vi "GUI_update.vi"(0 "reference":refnum<class "OSA.lvclass">, 5 "error in (no error)":errorcluster, 6 "ctrl refs":T1, 7 "y unit":T3, 9 "spectrum x unit":T2) -> (10 "acq stopped":bool, 14 "duplicate reference":refnum<class "OSA.lvclass">, 15 "X interferogram":cluster{"A":dbl, "B":dbl, "B-A":dbl} {"B-A" format="%^.2e"; "B" format="%.2f"; "A" format="%.2f"}, 16 "Y interferogram":cluster{"A":dbl, "B":dbl, "B-A":dbl} {"B-A" format="%^.2e"; "B" format="%.2f"; "A" format="%.2f"}, 17 "X spectrum":cluster{"A":dbl, "B":dbl, "B-A":dbl} {"B-A" format="%^.2e"; "B" format="%.2f"; "A" format="%.2f"}, 18 "Y spectrum":cluster{"A":dbl, "B":dbl, "B-A":dbl} {"B-A" format="%^.2e"; "B" format="%.2f"; "A" format="%.2f"}, 19 "error out":errorcluster)   [LabVIEW 2010, in "OSA.lvclass"]
doc: "Reads the contents of a <B>Thorlabs_OSA_64</B> object.\n\n[GOOP 1.0]"
uses:
  OSA.lvclass
  y_unit_GUI.ctl
  typeDef/spectrum_x_unit.ctl
  ctrlRefs.ctl
  typeDef/acq_dataType.ctl
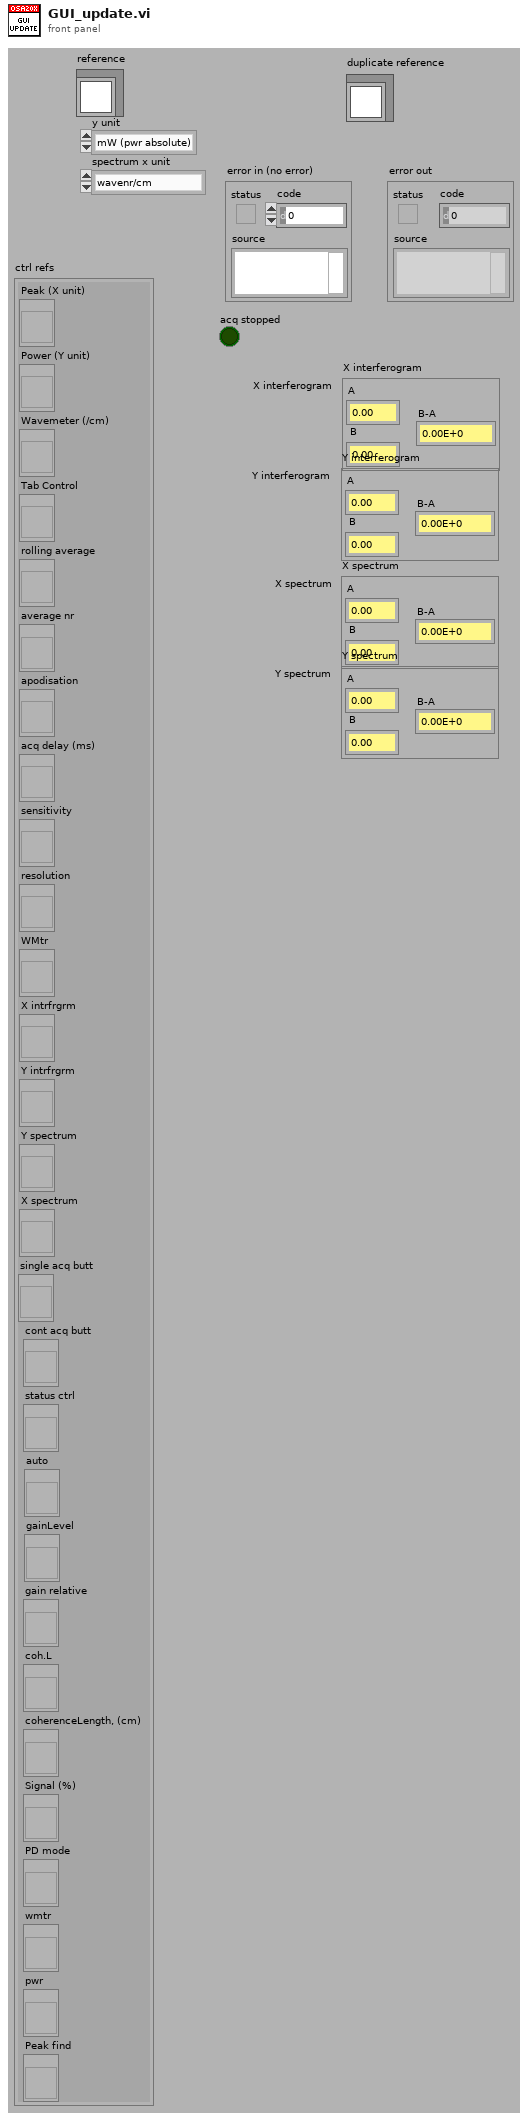
[diagram p1: front panel]
types:
  T1 = typedef "OSA.lvclass/ctrlRefs.ctl" = cluster{"Peak (X unit)":refnum<vi>, "Power (Y unit)":refnum<vi>, "Wavemeter (/cm)":refnum<vi>, "Tab Control":refnum<vi>, "rolling average":refnum<vi>, "average nr":refnum<vi>, "apodisation":refnum<vi>, "acq delay (ms)":refnum<vi>, "sensitivity":refnum<vi>, "resolution":refnum<vi>, "WMtr":refnum<vi>, "X intrfrgrm":refnum<vi>, "Y intrfrgrm":refnum<vi>, "Y spectrum":refnum<vi>, "X spectrum":refnum<vi>, "single acq butt":refnum<vi>, "cont acq butt":refnum<vi>, "status ctrl":refnum<vi>, "auto":refnum<vi>, "gainLevel":refnum<vi>, "gain relative":refnum<vi>, "coh.L":refnum<vi>, "coherenceLength, (cm)":refnum<vi>, "Signal (%)":refnum<vi>, "PD mode":refnum<vi>, "wmtr":refnum<vi>, "pwr":refnum<vi>, "Peak find":refnum<vi>}
  T2 = typedef "OSA.lvclass/spectrum_x_unit.ctl" = enum16{"wavenr/cm", "THz", "eV", "nm_air", "nm_vac"}
  T3 = typedef "OSA.lvclass/y_unit_GUI.ctl" = enum16{"mW (pwr absolute)", "dBm (pwr absolute)"}
  T4 = enum8{"Enabled", "Disabled", "Disabled and Grayed Out"}
  T5 = enum16{"cool: better sensitivity/noise floor", "warm: extended wl range"}
  T6 = typedef "OSA.lvclass/acq_dataType.ctl" = enum16{"none", "interferogram", "spectrum"}
  T7 = typedef "OSA.lvclass/ObjectAttributes.ctl" = cluster{"Stop":bool, "dataType":T6, "spectrometerIdx":u16, "buffer size interferogram":i32, "interferogram":cluster{"new":bool, "plot_x_ min":sgl, "plot_x_max":sgl, "plot_y_min":sgl, "plot_y_max":sgl, "Graph Intrfrgrm":T8, "timeStamp":u32, "signal (%)":dbl, "traces":cluster{"idx":u32, "broadBand":bool, "monoChromatic":bool, "peakToPeakSignal":dbl, "peakToPeakPos":dbl}[], "traces idx last":i32}, "spectrum":cluster{"new":bool, "plot_x_min":sgl, "plot_x_max":sgl, "plot_unit_x":T2, "plot_unit_y":T9, "plot_y_min":sgl, "plot_y_max":sgl, "Graph Spectrum":T8, "timeStamp":u32, "X_VAL_OPTIONS":enum16{"MIN_MAX", "ARRAY"}, "traces":cluster{"idx":u32}[], "traces idx last":i32}, "Thorlabs_OSA_64.lvclass:queue_action.ctlqueue ref":refnum<queue>, "action":T10, "plot zoom step":dbl, "buffer semaphore":T11, "acq stopped":bool, "dataType active":T6, "temperature (degr C)":sgl, "pressure (hPa)":sgl, "rel humidity (%)":sgl, "settings":cluster{"resolution":T12, "sensitivity":T13, "Average":bool, "average nr":u32, "apodisation":T14, "acq delay (ms)":u32, "airMesure":T15, "wmtr on":bool, "intfgrm_smooth_width":u16, "intfgrm_smooth_nrOfPasses":u16, "intfgrm_smooth":T16, "phaseCorrection":T17, "zeroFill":u8, "spectr_smooth":T16, "spectr_smooth_width":u16, "spectr_smooth_nrOfPasses":u16, "resolution (/cm)":sgl, "REF wavelength, (nm)":dbl, "gain_idx":u16, "gainAuto":bool, "gain_relative":dbl, "PD sensitivity mode":T18, "PD senseMode implemented":bool, "SensorTemperature implemented":bool, "SensorPressure implemented":bool, "SensorHumidity implemented":bool}, "peaks position":sgl[], "peaks width":sgl[], "peaks height":sgl[], "peaks max nr":u32, "peaks latest nr":i32, "peaks new":bool, "power":dbl, "power new":bool, "path":string, "wavelength (WNr)":dbl, "wavelength new":bool, "buffer size spectrum":i32, "status":string, "VI reference":refnum<vi>, "funcPointer":u64, "libraryPointer":u64, "singleAcquisition":bool, "coherenceLength (cm)":dbl, "coherenceLength new":bool, "spectrometer model":string, "spectrometer serial nr":string, "peaks thld left":sgl[], "peaks thld right":sgl[], "coherenceLength error (cm)":dbl, "ADC bits":u16, "peaks position centroid":sgl[], "peaks height centroid":sgl[], "OSA series":T19, "channel index":u16}
  T8 = typedef "OSA.lvclass/graph_intensity.ctl" = refnum<vi>
  T9 = typedef "OSA.lvclass/y_unit.ctl" = enum16{"ADC counts", "dBm pwr absolute", "dBm pwr density", "mW pwr absolute", "mW pwr density"}
  T10 = typedef "OSA.lvclass/queue_action.ctl" = enum16{"none", "stop", "GUI_plotInterferogram", "GUI_plotSpectrum", "GUI_plotInterferogramRescale", "GUI_plotSpectrumRescale", "GUI_plotInterferogramReset", "GUI_plotSpectrumReset", "GUI_plotInterferogramAutoScaleY", "GUI_plotSpectrumAutoScaleY", "GUI_plotInterferogramZoomOut", "GUI_plotSpectrumZoomOut", "GUI_plotInterferogramPane", "GUI_plotSpectrumPane", "GUI_plotInterferogramZoomMouse", "GUI_plotSpectrumZoomMouse", "ENVIRONMENT temperature", "ENVIRONMENT pressure", "MODE_resolution set", "MODE_resolution get", "MODE_sensitivity set", "MODE_sensitivity get", "MODE_PDTemperature set", "MODE_PDTemperature get", "REBOOT/RESET firmware", "ACQASYNC_acquireSingleSpectrum", "ACQASYNC_continuous start", "ACQASYNC_continuous stop\n", "ACQASYNC_get last interferogram", "ACQASYNC_get last spectrum", "ACQASYNC_get last waveNr", "ACQOPT_interferogram smoothing set", "ACQOPT_interferogram smoothing get", "ACQOPT_spectrum smoothing set", "ACQOPT_spectrum smoothing get", "ACQOPT_apodisation type set", "ACQOPT_apodisation type get", "ACQOPT_phase correction type set", "ACQOPT_phase correction type get", "ACQOPT_acqIntervall_set", "ACQOPT_acqIntervall_get", "ACQOPT_average spectrum set", "ACQOPT_average spectrum get", "ACQOPT_rolling average set", "ACQOPT_rolling average get", "ACQOPT_zero fill factor set", "ACQOPT_zero fill factor get", "ACQOPT_cycle counting set", "ACQOPT_cycle counting get", "ACQOPT_air measure option set", "ACQOPT_air measure option get", "ACQOPT_gainLevel auto get", "ACQOPT_gainLevel auto set", "ACQOPT_gainLevel get", "ACQOPT_gainLevel set", "ACQOPT_getAll", "INSTRUMENT_PROPERTY_range_WaveNr_min", "INSTRUMENT_PROPERTY_range_WaveNr_max", "INSTRUMENT_PROPERTY_reference_wavelength_cm^-1", "INSTRUMENT_PROPERTY_samplesPerRefPeriod", "INSTRUMENT_PROPERTY_resolution_waveNrPercm", "INSTRUMENT_PROPERTY_availableGainLevels", "INSTRUMENT_PROPERTY_status", "CONVERT", "ANALYSE_POWER", "ANALYSE_PEAKS", "ANALYSE_WAVELENGTH", "ANALYSE_SPECTRUM", "ANALYSE_INTERFEROGRAM", "ANALYSE_COHERENCE_LENGTH", "MATH", "MATH_power", "MATH_peaks", "FILE", "miscellaneous"}
  T11 = typedef "Semaphore RefNum" = refnum<k1>
  T12 = typedef "OSA.lvclass/resolution.ctl" = enum16{"low", "high"}
  T13 = typedef "OSA.lvclass/sensitivityMode.ctl" = enum16{"low", "low medium", "high medium", "high"}
  T14 = typedef "OSA.lvclass/apodisation.ctl" = enum16{"NONE", "NORTON_BEER_WEAK", "NORTON_BEER_MEDIUM", "NORTON_BEER_STRONG", "TRIANGULAR", "COSINE", "HANN", "HAMMING", "BLACKMANHARRIS3", "BLACKMANHARRIS4", "GAUSSIAN"}
  T15 = typedef "OSA.lvclass/airMeasure.ctl" = enum16{"TEMPERATURE", "PRESSURE"}
  T16 = typedef "OSA.lvclass/smoothing.ctl" = enum16{"NONE", "BINOMIAL", "SAVITSKY_GOLAY", "FOURIER", "MOVING_AVERAGE", "GAUSSIAN"}
  T17 = typedef "OSA.lvclass/phaseCorrection.ctl" = enum16{"NONE", "MERTZ", "FORMAN", "MERTZ_FILE", "FORMAN_FILE", "FUTURE COMP."}
  T18 = typedef "OSA.lvclass/PDTemperatureMode.ctl" = enum16{"cool: better sensitivity/noise floor", "warm: extended wl range"}
  T19 = typedef "OSA.lvclass/OSA_series.ctl" = enum16{"OSA200", "OSA300", "UNKNOWN"}
  T20 = typedef "Arrow Up.ctl" = bool
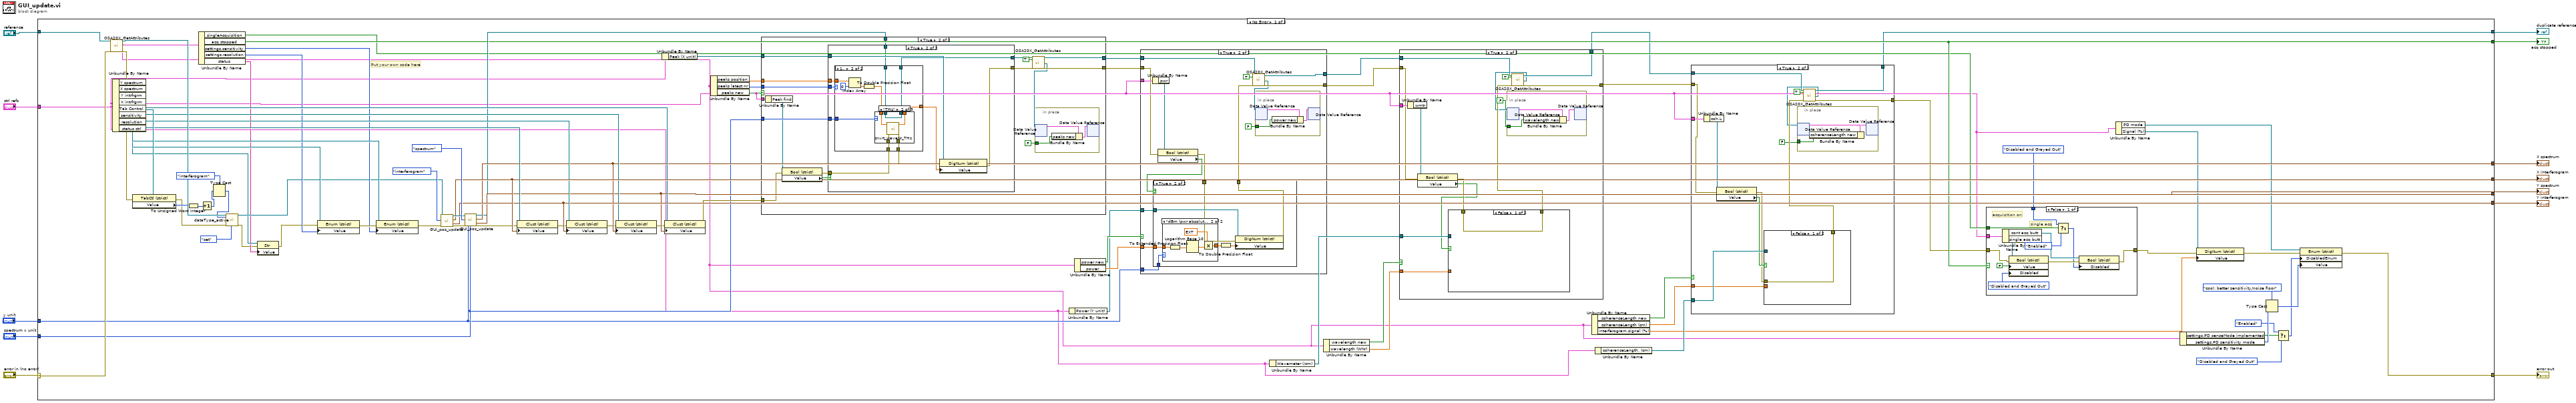
[diagram p0: block diagram]
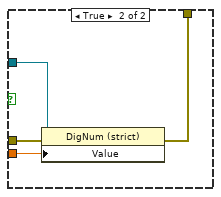
[diagram p3: hidden frame]
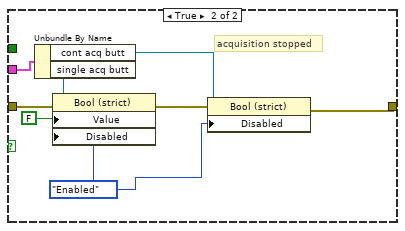
[diagram p4: hidden frame]
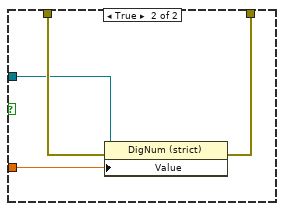
[diagram p6: hidden frame]
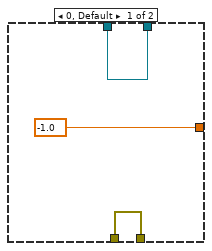
[diagram p12: hidden frame]
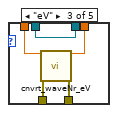
[diagram p14: hidden frame]
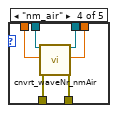
[diagram p15: hidden frame]
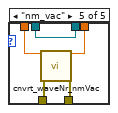
[diagram p16: hidden frame]
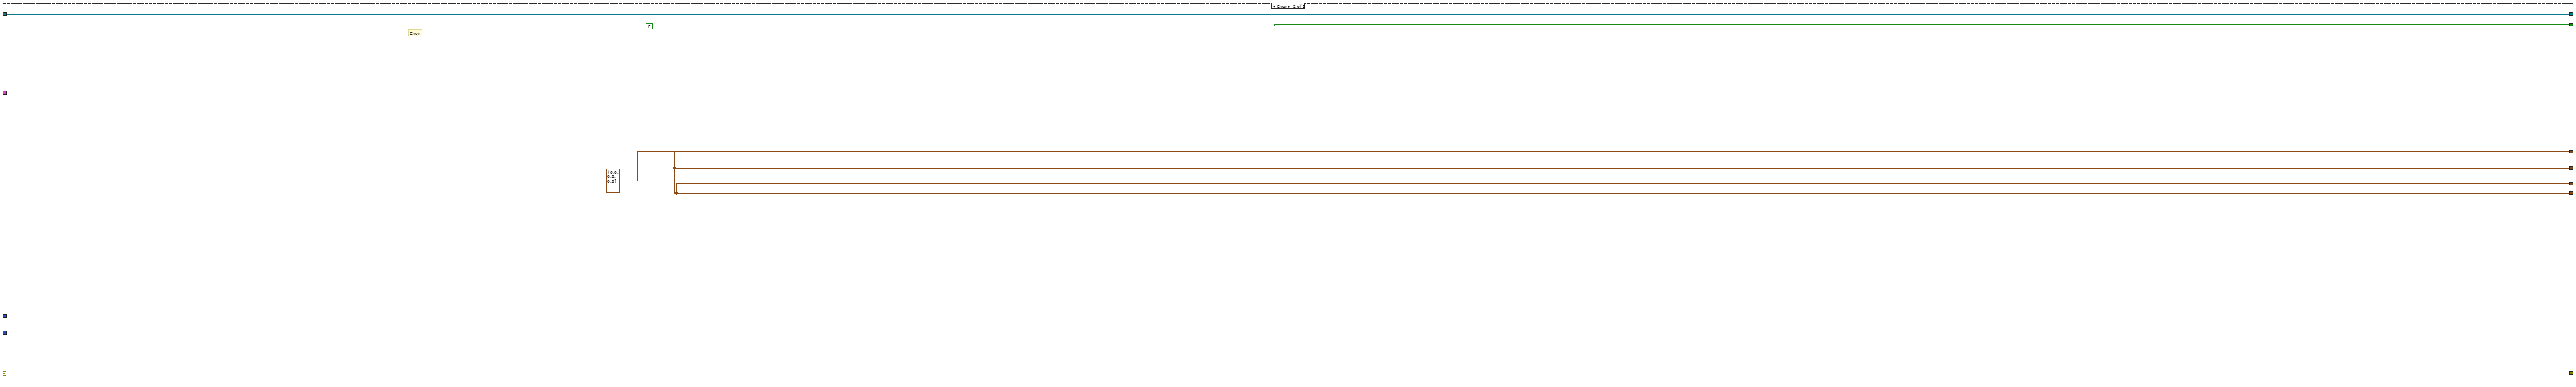
[diagram p17: hidden frame]
diagram:
  n1 = case shown="No Error" "error in (no error)" {
    selector: "error in (no error)" -> [w89 w270]
    tunnel: [w14 w270] -> w12
    tunnel: "reference" -> [w90 w271]
    tunnel: [w29 w271] -> w9
    tunnel: [w82 w269] -> w8
    tunnel: [w80 w269] -> w7
    tunnel: [w74 w269] -> w6
    tunnel: [w76 w269] -> w5
    tunnel: "spectrum x unit" -> [w58 _]
    tunnel: "y unit" -> [w50 _]
    tunnel: [w44 FALSE ("acq stopped")] -> w2
    tunnel: "ctrl refs" -> [w13 _]
    frame No Error {
      # "Put your own code here"
      n2 = call "OSA20X_GetAttributes.vi"("reference in"=w90, "error in (no error)"=w89) -> ("reference out"=w88:refnum<class "OSA.lvclass">, "Data"=w24:T7, "error out"=w71:errorcluster)  [unwired: 14 in, 1 out]
      n3 = Unbundle By Name(w13) -> ("Y spectrum"=w77:refnum<vi>, "X spectrum"=w78:refnum<vi>, "Y intrfrgrm"=w81:refnum<vi>, "X intrfrgrm"=w83:refnum<vi>, "Tab Control"=w84:refnum<vi>, "sensitivity"=w68:refnum<vi>, "resolution"=w67:refnum<vi>, "status ctrl"=w43:refnum<vi>)
      n4 = property class="TabCtl (strict)"(reference=w84, error in=w71) -> (error out=w85:errorcluster, "Value"=w87:enum32{"interferogram", "spectrum"})  [unwired: 1 out]
      n5 = To Unsigned Word Integer(number=w87) -> (unsigned 16bit integer=w86:u16)
      n6 = Unbundle By Name(w24) -> ("singleAcquisition"=w39:bool, "acq stopped"=w44:bool, "settings.sensitivity"=w65:T13, "settings.resolution"=w66:T12, "status"=w42:string)
      n7 = Increment(x=w86) -> (x+1=w36:u16)
      n8 = Type Cast(type=acq_dataType."interferogram" ("dataType active"), x=w36) -> (*(type *) &x=w35:T6)
      n9 = call "dataType_active.vi"("reference"=w88, "dataType active"=w35, "error in (no error)"=w85, "get/set"=enum16{"get", "set"}."set") -> ("duplicate reference"=w51:refnum<class "OSA.lvclass">, "error out"=w41:errorcluster)  [unwired: 13 in, 1 out]
      n10 = property class="Str"(reference=w43, error in=w41, "Value"=w42) -> (error out=w40:errorcluster)  [unwired: 1 out]
      n11 = property class="Enum (strict)"(reference=w67, error in=w40, "Value"=w66) -> (error out=w70:errorcluster)  [unwired: 1 out]
      n12 = property class="Enum (strict)"(reference=w68, error in=w70, "Value"=w65) -> (error out=w69:errorcluster)  [unwired: 1 out]
      n13 = call "GUI_pos_update.vi"("reference"=w51, "dataType"=acq_dataType."interferogram", "error in (no error)"=w69) -> ("reference out"=w92:refnum<class "OSA.lvclass">, "X"=w82:cluster{"A":dbl, "B":dbl, "B-A":dbl}, "Y"=w80:cluster{"A":dbl, "B":dbl, "B-A":dbl}, "error out"=w91:errorcluster)  [unwired: 13 in]
      n14 = call "GUI_pos_update.vi"("reference"=w92, "dataType"=acq_dataType."spectrum", "error in (no error)"=w91, "spectrum y unit"=w50, "spectrum x unit"=w58) -> ("reference out"=w59:refnum<class "OSA.lvclass">, "X"=w76:cluster{"A":dbl, "B":dbl, "B-A":dbl}, "Y"=w74:cluster{"A":dbl, "B":dbl, "B-A":dbl}, "error out"=w72:errorcluster)  [unwired: 11 in]
      n15 = property class="Clust (strict)"(reference=w83, error in=w72, "Value"=w82) -> (error out=w79:errorcluster)  [unwired: 1 out]
      n16 = property class="Clust (strict)"(reference=w81, error in=w79, "Value"=w80) -> (error out=w75:errorcluster)  [unwired: 1 out]
      n17 = property class="Clust (strict)"(reference=w78, error in=w75, "Value"=w76) -> (error out=w73:errorcluster)  [unwired: 1 out]
      n18 = Unbundle By Name(w13) -> ("Peak (X unit)"=w62:refnum<vi>)
      n19 = property class="Clust (strict)"(reference=w77, error in=w73, "Value"=w74) -> (error out=w64:errorcluster)  [unwired: 1 out]
      n20 = Unbundle By Name(w24) -> ("peaks position"=w60:sgl[], "peaks latest nr"=w61:i32, "peaks new"=w63:bool)
      n21 = case shown="True" w63 {
        tunnel: w64 -> [w197 w201]
        tunnel: w62 -> [_ w213]
        tunnel: w61 -> [_ w215]
        tunnel: w60 -> [_ w214]
        tunnel: [w197 w211] -> w52
        tunnel: w59 -> [w198 w205]
        tunnel: [w198 w210] -> w54
        tunnel: w58 -> [_ w209]
        tunnel: w13 -> [_ w203]
        frame False {
        }
        frame True {
          n22 = Unbundle By Name(w203) -> ("Peak find"=w202:refnum<vi>)
          n23 = property class="Bool (strict)"(reference=w202, error in=w201) -> (error out=w199:errorcluster, "Value"=w200:T20)  [unwired: 1 out]
          n24 = case shown="True" w200 {
            tunnel: w215 -> [_ w227]
            tunnel: w214 -> [_ w226]
            tunnel: w213 -> [_ w225]
            tunnel: [w216 w223] -> w212
            tunnel: w209 -> [_ w222]
            tunnel: w205 -> [w217 w221]
            tunnel: [w217 w220] -> w204
            tunnel: w199 -> [w216 w219]
            frame False {
            }
            frame True {
              n25 = case shown="1.." w227 {
                tunnel: w226 -> [_ w240]
                tunnel: [-1.0 ("Value") w237] -> w224
                tunnel: w222 -> [_ w236]
                tunnel: w219 -> [w229 w235]
                tunnel: [w229 w234] -> w218
                tunnel: w221 -> [w228 w233]
                tunnel: [w228 w232] -> w220
                frame 0, Default {
                }
                frame 1.. {
                  n26 = Index Array(array=w240, index=0) -> (element=w238:sgl)
                  n27 = To Double Precision Float(number=w238) -> (double precision float=w231:dbl)
                  n28 = case shown="\"THz\"" w236 {
                    tunnel: w231 -> [w241 w248 w253 w254 w264]
                    tunnel: [w241 w245 w250 w255 w261] -> w237
                    tunnel: w235 -> [w243 w247 w252 w259 w263]
                    tunnel: [w243 w246 w251 w258 w262] -> w234
                    tunnel: w233 -> [w242 w244 w249 w257 w260]
                    tunnel: [w242 w244 w249 w256 w260] -> w232
                    frame "wavenr/cm", Default {
                    }
                    frame "THz" {
                      n29 = call "cnvrt_waveNr_THz.vi"("waveNr"=w248, "error in (no error)"=w247) -> ("frequency (THz)"=w245:dbl, "error out"=w246:errorcluster)  [unwired: 16 in]
                    }
                    frame "eV" {
                      n30 = call "cnvrt_waveNr_eV.vi"("waveNr"=w253, "error in (no error)"=w252) -> ("energy (eV)"=w250:dbl, "error out"=w251:errorcluster)  [unwired: 16 in]
                    }
                    frame "nm_air" {
                      n31 = call "cnvrt_waveNr_nmAir.vi"("reference in"=w257, "waveNr"=w254, "error in (no error)"=w259) -> ("reference out"=w256:refnum<class "OSA.lvclass">, "wavelength (nmAir)"=w255:dbl, "error out"=w258:errorcluster)  [unwired: 14 in]
                    }
                    frame "nm_vac" {
                      n32 = call "cnvrt_waveNr_nmVac.vi"("waveNr"=w264, "error in (no error)"=w263) -> ("wavelength (nmVac)"=w261:dbl, "error out"=w262:errorcluster)  [unwired: 16 in]
                    }
                  }
                }
              }
              n33 = property class="DigNum (strict)"(reference=w225, error in=w218, "Value"=w224) -> (error out=w223:errorcluster)  [unwired: 1 out]
            }
          }
          n34 = call "OSA20X_GetAttributes.vi"("reference in"=w204, "OnlyGetDvrReference(False)"=TRUE, "error in (no error)"=w212) -> ("reference out"=w210:refnum<class "OSA.lvclass">, "DataRef"=w207:refnum<data-value>, "error out"=w211:errorcluster)  [unwired: 13 in, 1 out]
          n35 = in-place {
            in-place-border: FALSE ("peaks new") -> [w266]
            n36 = in-place-dvr #1(w207) -> (w267:T7)  [unwired: 1 out]
            n37 = Bundle By Name(cluster=w267, "peaks new"=w266) -> (w265:T7)
            n38 = in-place-dvr #1(w265) -> ()  [unwired: 2 out]
          }
        }
      }
      n39 = Unbundle By Name(w13) -> ("Power (Y unit)"=w53:refnum<vi>)
      n40 = Unbundle By Name(w24) -> ("power new"=w56:bool, "power"=w55:dbl)
      n41 = case shown="True" w56 {
        tunnel: w55 -> [_ w177]
        tunnel: w54 -> [w163 w179]
        tunnel: w53 -> [_ w178]
        tunnel: w52 -> [w164 w167]
        tunnel: [w164 w175] -> w45
        tunnel: w50 -> [_ w174]
        tunnel: [w163 w173] -> w46
        tunnel: w13 -> [_ w168]
        frame False {
        }
        frame True {
          n42 = Unbundle By Name(w168) -> ("pwr"=w169:refnum<vi>)
          n43 = property class="Bool (strict)"(reference=w169, error in=w167) -> (error out=w166:errorcluster, "Value"=w165:T20)  [unwired: 1 out]
          n44 = case shown="True" w165 {
            tunnel: w178 -> [_ w187]
            tunnel: w177 -> [_ w186]
            tunnel: [w180 w184] -> w176
            tunnel: w174 -> [_ w183]
            tunnel: w166 -> [w180 w181]
            frame False {
            }
            frame True {
              n45 = case shown="\"dBm (pwr absolute)\"" w183 {
                tunnel: w186 -> [w188 w191]
                tunnel: [w188 w192] -> w185
                frame "mW (pwr absolute)", Default {
                }
                frame "dBm (pwr absolute)" {
                  n46 = To Extended Precision Float(1:w191) -> (0:w190:ext)
                  n47 = Logarithm Base 10(1:w190) -> (0:w193:ext)
                  n48 = Multiply(x=ext 10.0, y=w193) -> (x*y=w192:ext)
                }
              }
              n49 = To Double Precision Float(number=w185) -> (double precision float=w182:dbl)
              n50 = property class="DigNum (strict)"(reference=w187, error in=w181, "Value"=w182) -> (error out=w184:errorcluster)  [unwired: 1 out]
            }
          }
          n51 = call "OSA20X_GetAttributes.vi"("reference in"=w179, "OnlyGetDvrReference(False)"=TRUE, "error in (no error)"=w176) -> ("reference out"=w173:refnum<class "OSA.lvclass">, "DataRef"=w171:refnum<data-value>, "error out"=w175:errorcluster)  [unwired: 13 in, 1 out]
          n52 = in-place {
            in-place-border: FALSE ("peaks new") -> [w195]
            n53 = in-place-dvr #2(w171) -> (w196:T7)  [unwired: 1 out]
            n54 = Bundle By Name(cluster=w196, "power new"=w195) -> (w194:T7)
            n55 = in-place-dvr #2(w194) -> ()  [unwired: 2 out]
          }
        }
      }
      n56 = Unbundle By Name(w13) -> ("Wavemeter (/cm)"=w47:refnum<vi>)
      n57 = Unbundle By Name(w24) -> ("wavelength new"=w49:bool, "wavelength (WNr)"=w48:dbl)
      n58 = case shown="True" w49 {
        tunnel: w48 -> [_ w152]
        tunnel: w46 -> [w139 w154]
        tunnel: w47 -> [_ w153]
        tunnel: w45 -> [w140 w143]
        tunnel: [w140 w150] -> w31
        tunnel: [w139 w149] -> w30
        tunnel: w13 -> [_ w144]
        frame False {
        }
        frame True {
          n59 = Unbundle By Name(w144) -> ("wmtr"=w145:refnum<vi>)
          n60 = property class="Bool (strict)"(reference=w145, error in=w143) -> (error out=w142:errorcluster, "Value"=w141:T20)  [unwired: 1 out]
          n61 = case shown="False" w141 {
            tunnel: w142 -> [w155 w159]
            tunnel: w153 -> [_ w158]
            tunnel: w152 -> [_ w157]
            tunnel: [w155 w156] -> w151
            frame False {
            }
            frame True {
              n62 = property class="DigNum (strict)"(reference=w158, error in=w159, "Value"=w157) -> (error out=w156:errorcluster)  [unwired: 1 out]
            }
          }
          n63 = call "OSA20X_GetAttributes.vi"("reference in"=w154, "OnlyGetDvrReference(False)"=TRUE, "error in (no error)"=w151) -> ("reference out"=w149:refnum<class "OSA.lvclass">, "DataRef"=w147:refnum<data-value>, "error out"=w150:errorcluster)  [unwired: 13 in, 1 out]
          n64 = in-place {
            in-place-border: FALSE ("peaks new") -> [w161]
            n65 = in-place-dvr #3(w147) -> (w162:T7)  [unwired: 1 out]
            n66 = Bundle By Name(cluster=w162, "wavelength new"=w161) -> (w160:T7)
            n67 = in-place-dvr #3(w160) -> ()  [unwired: 2 out]
          }
        }
      }
      n68 = Unbundle By Name(w24) -> ("coherenceLength new"=w34:bool, "coherenceLength (cm)"=w33:dbl, "interferogram.signal (%)"=w26:dbl)
      n69 = Unbundle By Name(w13) -> ("coherenceLength, (cm)"=w32:refnum<vi>)
      n70 = case shown="True" w34 {
        tunnel: w33 -> [_ w108]
        tunnel: w30 -> [w95 w110]
        tunnel: w32 -> [_ w109]
        tunnel: w31 -> [w96 w98]
        tunnel: [w96 w106] -> w28
        tunnel: [w95 w105] -> w29
        tunnel: w13 -> [_ w100]
        frame False {
        }
        frame True {
          n71 = Unbundle By Name(w100) -> ("coh.L"=w101:refnum<vi>)
          n72 = property class="Bool (strict)"(reference=w101, error in=w98) -> (error out=w97:errorcluster, "Value"=w99:T20)  [unwired: 1 out]
          n73 = case shown="False" w99 {
            tunnel: w97 -> [w111 w115]
            tunnel: w109 -> [_ w114]
            tunnel: w108 -> [_ w113]
            tunnel: [w111 w112] -> w107
            frame False {
            }
            frame True {
              n74 = property class="DigNum (strict)"(reference=w114, error in=w115, "Value"=w113) -> (error out=w112:errorcluster)  [unwired: 1 out]
            }
          }
          n75 = call "OSA20X_GetAttributes.vi"("reference in"=w110, "OnlyGetDvrReference(False)"=TRUE, "error in (no error)"=w107) -> ("reference out"=w105:refnum<class "OSA.lvclass">, "DataRef"=w103:refnum<data-value>, "error out"=w106:errorcluster)  [unwired: 13 in, 1 out]
          n76 = in-place {
            in-place-border: FALSE ("peaks new") -> [w117]
            n77 = in-place-dvr #4(w103) -> (w118:T7)  [unwired: 1 out]
            n78 = Bundle By Name(cluster=w118, "coherenceLength new"=w117) -> (w116:T7)
            n79 = in-place-dvr #4(w116) -> ()  [unwired: 2 out]
          }
        }
      }
      n80 = case shown="False" w44 {
        tunnel: w13 -> [w127 w138]
        tunnel: w28 -> [w128 w137]
        tunnel: [w125 w132] -> w27
        tunnel: w39 -> [w123 _]
        tunnel: T4."Disabled and Grayed Out" ("Disabled") -> [w122 _]
        frame False {
          # "acquisition on"
          # "single acq"
          n81 = Unbundle By Name(w127) -> ("cont acq butt"=w124:refnum<vi>, "single acq butt"=w130:refnum<vi>)
          n82 = property class="Bool (strict)"(reference=w130, error in=w128, "Value"=FALSE, "Disabled"=T4."Disabled and Grayed Out") -> (error out=w126:errorcluster)  [unwired: 1 out]
          n83 = Select(t=w122, s=w123, f=T4."Enabled") -> (s? t:f=w120:T4)
          n84 = property class="Bool (strict)"(reference=w124, error in=w126, "Disabled"=w120) -> (error out=w125:errorcluster)  [unwired: 1 out]
        }
        frame True {
          w131 = T4."Enabled" ("Disabled")
          # "acquisition stopped"
          n85 = Unbundle By Name(w138) -> ("cont acq butt"=w133:refnum<vi>, "single acq butt"=w136:refnum<vi>)
          n86 = property class="Bool (strict)"(reference=w136, error in=w137, "Value"=FALSE, "Disabled"=w131) -> (error out=w134:errorcluster)  [unwired: 1 out]
          n87 = property class="Bool (strict)"(reference=w133, error in=w134, "Disabled"=w131) -> (error out=w132:errorcluster)  [unwired: 1 out]
        }
      }
      n88 = Unbundle By Name(w13) -> ("PD mode"=w22:refnum<vi>, "Signal (%)"=w25:refnum<vi>)
      n89 = Unbundle By Name(w24) -> ("settings.PD senseMode implemented"=w18:bool, "settings.PD sensitivity mode"=w20:T18)
      n90 = property class="DigNum (strict)"(reference=w25, error in=w27, "Value"=w26) -> (error out=w23:errorcluster)  [unwired: 1 out]
      n91 = Type Cast(type=T5."cool: better sensitivity/noise floor" ("Value"), x=w20) -> (*(type *) &x=w19:T5)
      n92 = Select(t=T4."Enabled" ("Disabled"), s=w18, f=T4."Disabled and Grayed Out") -> (s? t:f=w15:T4)
      n93 = property class="Enum (strict)"(reference=w22, error in=w23, "DisabledEnum"=w15, "Value"=w19) -> (error out=w14:errorcluster)  [unwired: 1 out]
    }
    frame Error {
      w269 = cluster{"A":dbl, "B":dbl, "B-A":dbl} {"A"=0.0, "B"=0.0, "B-A"=0.0} ("X")
      # "Error"
    }
  }
  "error out" <- w12
  "duplicate reference" <- w9
  "X interferogram" <- w8
  "Y interferogram" <- w7
  "Y spectrum" <- w6
  "X spectrum" <- w5
  "acq stopped" <- w2
